vi "ztscopeM Acquisition.vi"(6 "Trigger Mode":i32(ring) items=["Auto", "Normal"], 7 "Initiate Continuously":i32(ring) items=["Continuously"=1, "Single Capture"=0], 8 "error in":errorcluster, 9 "Acquire Count":i32=1, 10 "Acquire Type":i32(ring) items=["Normal"=0, "Average"=1, "Envelope"=2, "Peak Detect"=3, "High Resolution"=4, "Fast"=5, "Equivalent Time"=16], 11 "Instrument Handle In":i32) -> (0 "error out":errorcluster, 3 "Instrument Handle Out":i32)   [LabVIEW 2013]
doc: "Configure the acquisition settings."
uses:
  ztscopeM.dll
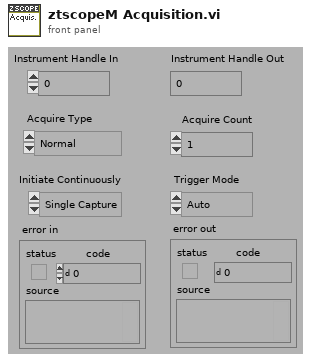
[diagram p1: front panel]
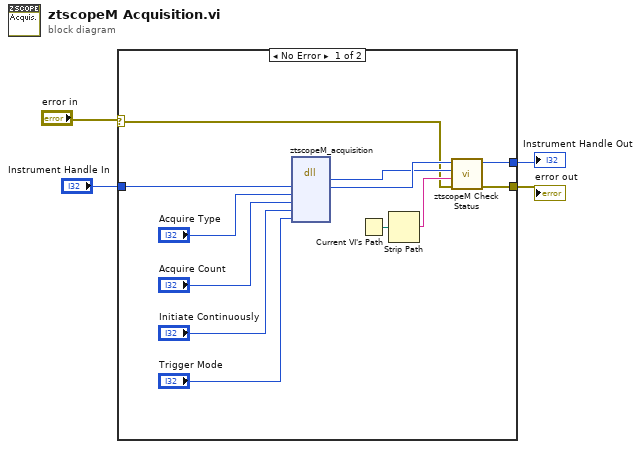
[diagram p0: block diagram]
diagram:
  n1 = case shown="No Error" "error in" {
    selector: "error in" -> [w7 w18]
    tunnel: [w6 w18] -> w1
    tunnel: "Instrument Handle In" -> [w16 w17]
    tunnel: [w5 w17] -> w3
    frame No Error {
      n2 = dll-call lib="C:/Program Files/National Instruments/instr.lib/ztscopem/ztscopeM.dll" fn="ztscopeM_acquisition"("instrumentHandle"=w16, "acquireType"="Acquire Type", "acquireCount"="Acquire Count", "initiateContinuously"="Initiate Continuously", "triggerMode"="Trigger Mode") -> (w8:i32, "instrumentHandle"=w9:i32)  [unwired: 7 in, 2 out]
      n3 = Current VI's Path() -> (path=w11:path)
      n4 = Strip Path(path=w11) -> (name=w10:string)  [unwired: 1 out]
      n5 = call "ztscopeM Check Status.vi"("error in"=w7, "name of VI"=w10, "status"=w8, "instrument handle in"=w9) -> ("error out"=w6:errorcluster, "instrument handle out"=w5:i32)  [unwired: 2 in]
    }
    frame Error {
    }
  }
  "Instrument Handle Out" <- w3
  "error out" <- w1
